vi "Write Bucket.vi"(8 "error in (no error)":errorcluster, 10 "Bucket":refnum<class "Bucket.lvclass">, 11 "Multipart Upload in":refnum<class "Multipart Upload.lvclass">) -> (0 "error out":errorcluster, 3 "Multipart Upload out":refnum<class "Multipart Upload.lvclass">)   [LabVIEW 2015, in "NI_AWS_S3.lvlib" / "Multipart Upload.lvclass"]
uses:
  Multipart Upload.lvclass
  Bucket/Bucket.lvclass
  Multipart Upload.lvclass/Multipart Upload.ctl
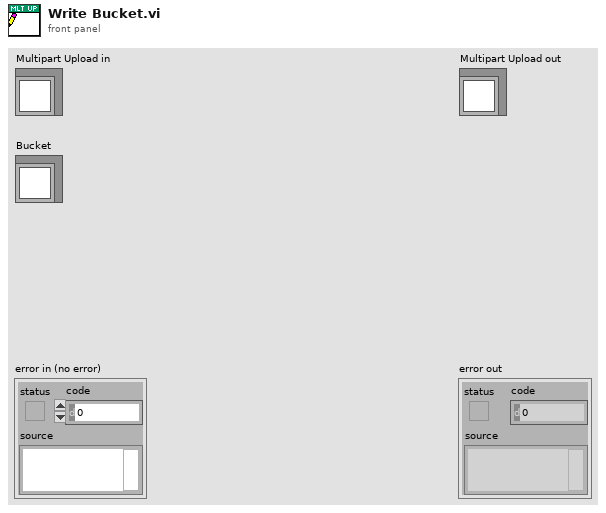
[diagram p1: front panel]
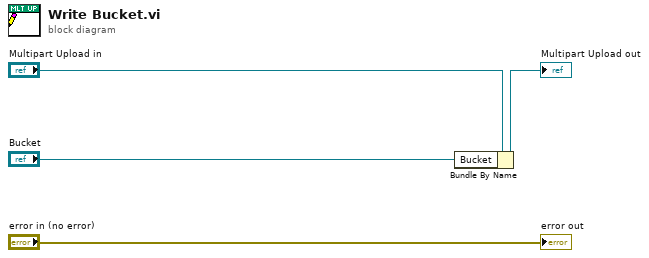
[diagram p0: block diagram]
diagram:
  n1 = Bundle By Name(cluster="Multipart Upload in", "Bucket"="Bucket") -> (→"Multipart Upload out":refnum<class "Multipart Upload.lvclass">)
  "error out" <- "error in (no error)"
